vi "VCS Export Channel Data To File.vi"(8 "error in (no error)":errorcluster, 9 "fileName":string, 11 "axis in":cluster{"keyHandle":u32, "nodeId":u16}={"keyHandle"=0, "nodeId"=1}) -> (0 "error out":errorcluster, 3 "axis out":cluster{"keyHandle":u32, "nodeId":u16}={"keyHandle"=0, "nodeId"=1})   [LabVIEW 2018]
doc: "<B>VCS_ExportChannelDataToFile</B> saves data point in a file (File endings: *.csv, *.txt or *.rda)."
uses:
  Resources/EposCmd.dll
  Resources/EposCmd64.dll
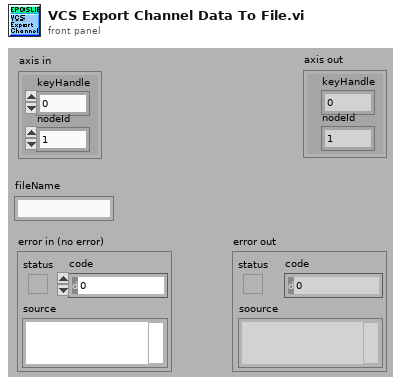
[diagram p1: front panel]
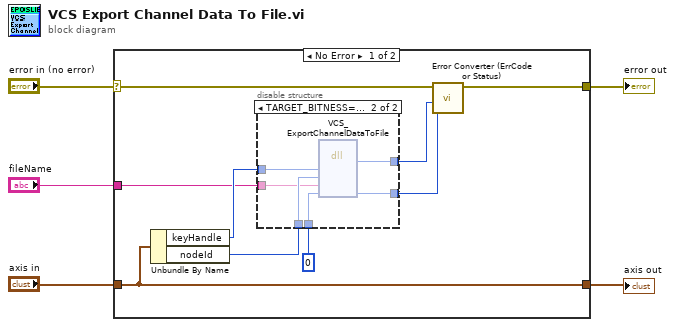
[diagram p0: block diagram]
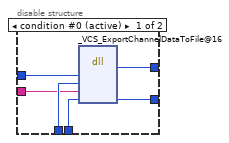
[diagram p2: hidden frame]
diagram:
  n1 = case shown="No Error" "error in (no error)" {
    selector: "error in (no error)" -> [w12 w27]
    tunnel: "axis in" -> [w14 w28]
    tunnel: [w14 w28] -> w4
    tunnel: [w13 w27] -> w3
    tunnel: "fileName" -> [w6 _]
    frame No Error {
      n2 = Unbundle By Name(w14) -> ("keyHandle"=w8:u32, "nodeId"=w7:u16)
      n3 = disable-structure shown="TARGET_BITNESS==64" {
        disable-tunnel: u32 0 ("pErrorCode") -> [w20 w26]
        disable-tunnel: [w19 w25] -> w10
        disable-tunnel: [w18 w24] -> w9
        disable-tunnel: w8 -> [w17 w23]
        disable-tunnel: w7 -> [w16 w22]
        disable-tunnel: w6 -> [w15 w21]
        frame condition #0 (active) {
          n4 = dll-call lib="C:/Projeto em LabVIEW/EPOS-LabVIEW-Instrument-Driver-En/LabVIEW/maxon EPOS/Resources/EposCmd.*" fn="_VCS_ExportChannelDataToFile@16"("KeyHandle"=w17, "NodeId"=w16, "FileName"=w15, "pErrorCode"=w20) -> (w18:i32, "pErrorCode"=w19:u32)  [unwired: 6 in, 2 out]
        }
        frame condition #1 {
          n5 = dll-call lib="C:/setup/Resources/EposCmd64.*" fn="VCS_ExportChannelDataToFile" ("EposCmd.dll:_VCS_ExportChannelDataToFile@16")("KeyHandle"=w23, "NodeId"=w22, "FileName"=w21, "pErrorCode"=w26) -> ("Rückgabetyp"=w24:i32, "pErrorCode"=w25:u32)  [unwired: 6 in, 2 out]
        }
      }
      n6 = call "Error Converter (ErrCode or Status).vi"("error code"=w10, "return type"=w9, "error in (no error)"=w12) -> ("error out"=w13:errorcluster)  [unwired: 7 in]
    }
    frame Error {
    }
  }
  "error out" <- w3
  "axis out" <- w4
